vi "Wield.vi"(8 "Error In":errorcluster, 11 "reference in":refnum<class "Sword.lvclass">) -> (0 "Error Out":errorcluster, 3 "reference out":refnum<class "Sword.lvclass">)   [LabVIEW 2020, in "Sword.lvclass"]
uses:
  Sword.lvclass
  IEnchantment_interface/IEnchantment.lvclass
  Console_class/Console.lvclass
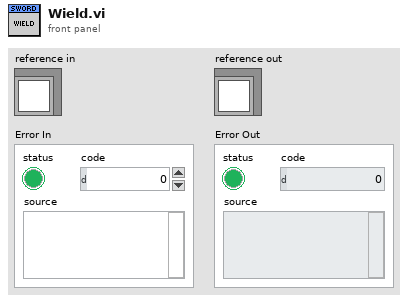
[diagram p1: front panel]
types:
  T1 = typedef "Sword.lvclass/ObjectAttributes.ctl" = cluster{"_enchantment":refnum<class "IEnchantment.lvclass">}
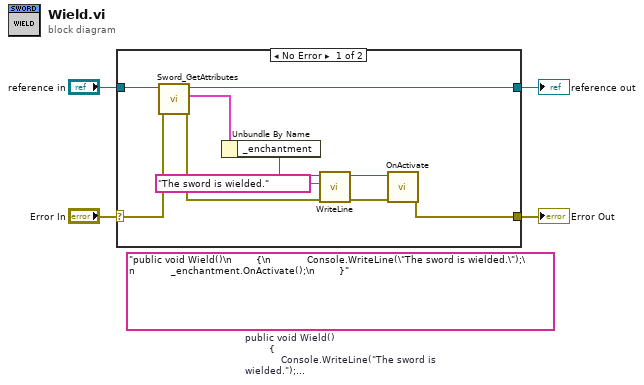
[diagram p0: block diagram]
diagram:
  (unwired) "public void Wield()\n        {\n            Console.WriteLine(\"The sword is wielded.\");\n            _enchantment.OnActivate();\n        }"  # public void Wield()         {             Console.WriteLine("The sword is wielded.");             _enchantment.OnActivate();         }
  n1 = case shown="No Error" "Error In" {
    selector: "Error In" -> [w12 w15]
    tunnel: [w5 w15] -> w3
    tunnel: [w11 w14] -> w1
    tunnel: "reference in" -> [w13 w14]
    frame No Error {
      n2 = call "Sword_GetAttributes.vi"("error in (no error)"=w12, "reference in"=w13) -> ("error out"=w8:errorcluster, "Data"=w10:T1, "reference out"=w11:refnum<class "Sword.lvclass">)  [unwired: 6 in, 1 out]
      n3 = Unbundle By Name(w10) -> ("_enchantment"=w9:refnum<class "IEnchantment.lvclass">)
      n4 = call "WriteLine.vi"("Error In"=w8, "ConsoleText"="The sword is wielded.") -> ("Error Out"=w6:errorcluster)  [unwired: 9 in]
      n5 = call-dynamic "OnActivate.vi"("Error In"=w6, "object in"=w9) -> ("Error Out"=w5:errorcluster)  [unwired: 8 in, 1 out]
    }
    frame Error {
    }
  }
  "Error Out" <- w3
  "reference out" <- w1
